vi "MICSD Config.vi"(8 "error in (no error)":errorcluster, 9 "Function":enum16{"Write Config", "Read Config"}(ring), 10 "MICS_Config_In":T1={"ConfigFlags"=0, "ImplantID"=1193046, "CompanyID"=1, "Normal_Comm"={"RF_Channel"=4, "UserData"=0, "TX_Mod"=0, "RX_Mod"=0, "RX_BlockSize"=15, "BlockPerPack"=31, "TX_BlockSize"=15}, "Emerg_Comm"={"RF_Channel"=4, "UserData"=0, "TX_Mod"=0, "RX_Mod"=0, "TX_BlockSize"=15, "BlockPerPack"=31, "RX_BlockSize"=15}, "ImplantRev"=5, "245TX_PowerCal"=0, "245TX_Power"=10, "CCA_RSSI_Thresholds"={"ch0"=2650, "ch1"=2650, "ch2"=2650, "ch3"=2650, "ch4"=2650, "ch5"=2650, "ch6"=2650, "ch7"=2650, "ch8"=2650, "ch9"=2650}} {"ConfigFlags" format="%02x"; "ImplantID" format="%06x"; "CompanyID" format="%02x"; "Normal_Comm"."TX_BlockSize" items=["2"=2, "3"=3, "4"=4, "5"=5, "6"=6, "7"=7, "8"=8, "9"=9, "10"=10, "11"=11, "12"=12, "13"=13, "14"=14, "15"=15, "16"=16, "17"=17, "18"=18, "19"=19, "20"=20, "21"=21, "22"=22, "23"=23, "24"=24, "25"=25, "26"=26, "27"=27, "28"=28, "29"=29, "30"=30, "31"=31]; "Normal_Comm"."RF_Channel" items=["0", "1", "2", "3", "4", "5", "6", "7", "8", "9", "10", "11"]; "Normal_Comm"."UserData" items=["0 - 000"=0, "1 - 001"=16, "2 - 010"=32, "3 - 011"=48, "4 - 100"=64, "5 - 101"=80, "6 - 110"=96, "7 - 111"=112]; "Normal_Comm"."TX_Mod" items=["2FSK-FB"=0, "2FSK"=2, "4FSK"=3]; "Normal_Comm"."RX_Mod" items=["2FSK-FB"=0, "2FSK"=8, "4FSK"=12]; "Normal_Comm"."RX_BlockSize" items=["2"=2, "3"=3, "4"=4, "5"=5, "6"=6, "7"=7, "8"=8, "9"=9, "10"=10, "11"=11, "12"=12, "13"=13, "14"=14, "15"=15, "16"=16, "17"=17, "18"=18, "19"=19, "20"=20, "21"=21, "22"=22, "23"=23, "24"=24, "25"=25, "26"=26, "27"=27, "28"=28, "29"=29, "30"=30, "31"=31]; "Normal_Comm"."BlockPerPack" items=["1"=1, "2"=2, "3"=3, "4"=4, "5"=5, "6"=6, "7"=7, "8"=8, "9"=9, "10"=10, "11"=11, "12"=12, "13"=13, "14"=14, "15"=15, "16"=16, "17"=17, "18"=18, "19"=19, "20"=20, "21"=21, "22"=22, "23"=23, "24"=24, "25"=25, "26"=26, "27"=27, "28"=28, "29"=29, "30"=30, "31"=31]; "Emerg_Comm"."RX_BlockSize" items=["2"=2, "3"=3, "4"=4, "5"=5, "6"=6, "7"=7, "8"=8, "9"=9, "10"=10, "11"=11, "12"=12, "13"=13, "14"=14, "15"=15, "16"=16, "17"=17, "18"=18, "19"=19, "20"=20, "21"=21, "22"=22, "23"=23, "24"=24, "25"=25, "26"=26, "27"=27, "28"=28, "29"=29, "30"=30, "31"=31]; "Emerg_Comm"."RF_Channel" items=["0", "1", "2", "3", "4", "5", "6", "7", "8", "9"]; "Emerg_Comm"."UserData" items=["0 - 000"=0, "1 - 001"=16, "2 - 010"=32, "3 - 011"=48, "4 - 100"=64, "5 - 101"=80, "6 - 110"=96, "7 - 111"=112]; "Emerg_Comm"."TX_Mod" items=["2FSK-FB"=0, "2FSK"=2, "4FSK"=3]; "Emerg_Comm"."RX_Mod" items=["2FSK-FB"=0, "2FSK"=8, "4FSK"=12]; "Emerg_Comm"."TX_BlockSize" items=["2"=2, "3"=3, "4"=4, "5"=5, "6"=6, "7"=7, "8"=8, "9"=9, "10"=10, "11"=11, "12"=12, "13"=13, "14"=14, "15"=15, "16"=16, "17"=17, "18"=18, "19"=19, "20"=20, "21"=21, "22"=22, "23"=23, "24"=24, "25"=25, "26"=26, "27"=27, "28"=28, "29"=29, "30"=30, "31"=31]; "Emerg_Comm"."BlockPerPack" items=["1"=1, "2"=2, "3"=3, "4"=4, "5"=5, "6"=6, "7"=7, "8"=8, "9"=9, "10"=10, "11"=11, "12"=12, "13"=13, "14"=14, "15"=15, "16"=16, "17"=17, "18"=18, "19"=19, "20"=20, "21"=21, "22"=22, "23"=23, "24"=24, "25"=25, "26"=26, "27"=27, "28"=28, "29"=29, "30"=30, "31"=31]; "ImplantRev" items=["ZL70100"=0, "ZL70101"=1, "ZL70102"=4, "ZL70103"=5]; "245TX_PowerCal" items=["-29"=-29, "-4"=-4, "-2"=-2, "0"=0, "2"=2, "4"=4, "6"=6, "8"=8, "10"=10, "12"=12, "14"=14, "16"=16, "18"=18, "20"=20, "22"=22, "24"=24, "26"=26, "27"=27]; "245TX_Power" items=["-29"=-29, "-4"=-4, "-2"=-2, "0"=0, "2"=2, "4"=4, "6"=6, "8"=8, "10"=10, "12"=12, "14"=14, "16"=16, "18"=18, "20"=20, "22"=22, "24"=24, "26"=26, "27"=27]}, 11 "VISA Resource Name":refnum<visa-resource-name>) -> (0 "error out":errorcluster, 1 "Reply Header":u8[](array[numeric]), 3 "dup VISA Resource Name":refnum<visa-resource-name>)   [LabVIEW 2020]
uses:
  <vilib>/Instr/_visa.llb/VISA Configure Serial Port (Instr).vi
panel:
  out "Written Config":u8[](array[numeric]) format="%02x"
  out "MICS_Config_OUT":T1={"ConfigFlags"=0, "ImplantID"=1048576, "CompanyID"=187, "Normal_Comm"={"RF_Channel"=4, "UserData"=0, "TX_Mod"=2, "RX_Mod"=8, "RX_BlockSize"=15, "BlockPerPack"=31, "TX_BlockSize"=15}, "Emerg_Comm"={"RF_Channel"=4, "UserData"=0, "TX_Mod"=2, "RX_Mod"=8, "TX_BlockSize"=15, "BlockPerPack"=31, "RX_BlockSize"=15}, "ImplantRev"=4, "245TX_PowerCal"=0, "245TX_Power"=10, "CCA_RSSI_Thresholds"={"ch0"=2650, "ch1"=2650, "ch2"=2650, "ch3"=2650, "ch4"=2650, "ch5"=2650, "ch6"=2650, "ch7"=2650, "ch8"=2650, "ch9"=2650}} {"ConfigFlags" format="%02x"; "ImplantID" format="%06x"; "CompanyID" format="%02x"; "Normal_Comm"."TX_BlockSize" items=["2"=2, "3"=3, "4"=4, "5"=5, "6"=6, "7"=7, "8"=8, "9"=9, "10"=10, "11"=11, "12"=12, "13"=13, "14"=14, "15"=15, "16"=16, "17"=17, "18"=18, "19"=19, "20"=20, "21"=21, "22"=22, "23"=23, "24"=24, "25"=25, "26"=26, "27"=27, "28"=28, "29"=29, "30"=30, "31"=31]; "Normal_Comm"."RF_Channel" items=["0", "1", "2", "3", "4", "5", "6", "7", "8", "9"]; "Normal_Comm"."UserData" items=["0 - 000"=0, "1 - 001"=16, "2 - 010"=32, "3 - 011"=48, "4 - 100"=64, "5 - 101"=80, "6 - 110"=96, "7 - 111"=112]; "Normal_Comm"."TX_Mod" items=["2FSK-FB"=0, "2FSK"=2, "4FSK"=3]; "Normal_Comm"."RX_Mod" items=["2FSK-FB"=0, "2FSK"=8, "4FSK"=12]; "Normal_Comm"."RX_BlockSize" items=["2"=2, "3"=3, "4"=4, "5"=5, "6"=6, "7"=7, "8"=8, "9"=9, "10"=10, "11"=11, "12"=12, "13"=13, "14"=14, "15"=15, "16"=16, "17"=17, "18"=18, "19"=19, "20"=20, "21"=21, "22"=22, "23"=23, "24"=24, "25"=25, "26"=26, "27"=27, "28"=28, "29"=29, "30"=30, "31"=31]; "Normal_Comm"."BlockPerPack" items=["1"=1, "2"=2, "3"=3, "4"=4, "5"=5, "6"=6, "7"=7, "8"=8, "9"=9, "10"=10, "11"=11, "12"=12, "13"=13, "14"=14, "15"=15, "16"=16, "17"=17, "18"=18, "19"=19, "20"=20, "21"=21, "22"=22, "23"=23, "24"=24, "25"=25, "26"=26, "27"=27, "28"=28, "29"=29, "30"=30, "31"=31]; "Emerg_Comm"."RX_BlockSize" items=["2"=2, "3"=3, "4"=4, "5"=5, "6"=6, "7"=7, "8"=8, "9"=9, "10"=10, "11"=11, "12"=12, "13"=13, "14"=14, "15"=15, "16"=16, "17"=17, "18"=18, "19"=19, "20"=20, "21"=21, "22"=22, "23"=23, "24"=24, "25"=25, "26"=26, "27"=27, "28"=28, "29"=29, "30"=30, "31"=31]; "Emerg_Comm"."RF_Channel" items=["0", "1", "2", "3", "4", "5", "6", "7", "8", "9"]; "Emerg_Comm"."UserData" items=["0 - 000"=0, "1 - 001"=16, "2 - 010"=32, "3 - 011"=48, "4 - 100"=64, "5 - 101"=80, "6 - 110"=96, "7 - 111"=112]; "Emerg_Comm"."TX_Mod" items=["2FSK-FB"=0, "2FSK"=2, "4FSK"=3]; "Emerg_Comm"."RX_Mod" items=["2FSK-FB"=0, "2FSK"=8, "4FSK"=12]; "Emerg_Comm"."TX_BlockSize" items=["2"=2, "3"=3, "4"=4, "5"=5, "6"=6, "7"=7, "8"=8, "9"=9, "10"=10, "11"=11, "12"=12, "13"=13, "14"=14, "15"=15, "16"=16, "17"=17, "18"=18, "19"=19, "20"=20, "21"=21, "22"=22, "23"=23, "24"=24, "25"=25, "26"=26, "27"=27, "28"=28, "29"=29, "30"=30, "31"=31]; "Emerg_Comm"."BlockPerPack" items=["1"=1, "2"=2, "3"=3, "4"=4, "5"=5, "6"=6, "7"=7, "8"=8, "9"=9, "10"=10, "11"=11, "12"=12, "13"=13, "14"=14, "15"=15, "16"=16, "17"=17, "18"=18, "19"=19, "20"=20, "21"=21, "22"=22, "23"=23, "24"=24, "25"=25, "26"=26, "27"=27, "28"=28, "29"=29, "30"=30, "31"=31]; "ImplantRev" items=["ZL70100"=0, "ZL70101"=1, "ZL70102"=4, "ZL70103"=5]; "245TX_PowerCal" items=["-29"=-29, "-4"=-4, "-2"=-2, "0"=0, "2"=2, "4"=4, "6"=6, "8"=8, "10"=10, "12"=12, "14"=14, "16"=16, "18"=18, "20"=20, "22"=22, "24"=24, "26"=26, "27"=27]; "245TX_Power" items=["-29"=-29, "-4"=-4, "-2"=-2, "0"=0, "2"=2, "4"=4, "6"=6, "8"=8, "10"=10, "12"=12, "14"=14, "16"=16, "18"=18, "20"=20, "22"=22, "24"=24, "26"=26, "27"=27]}
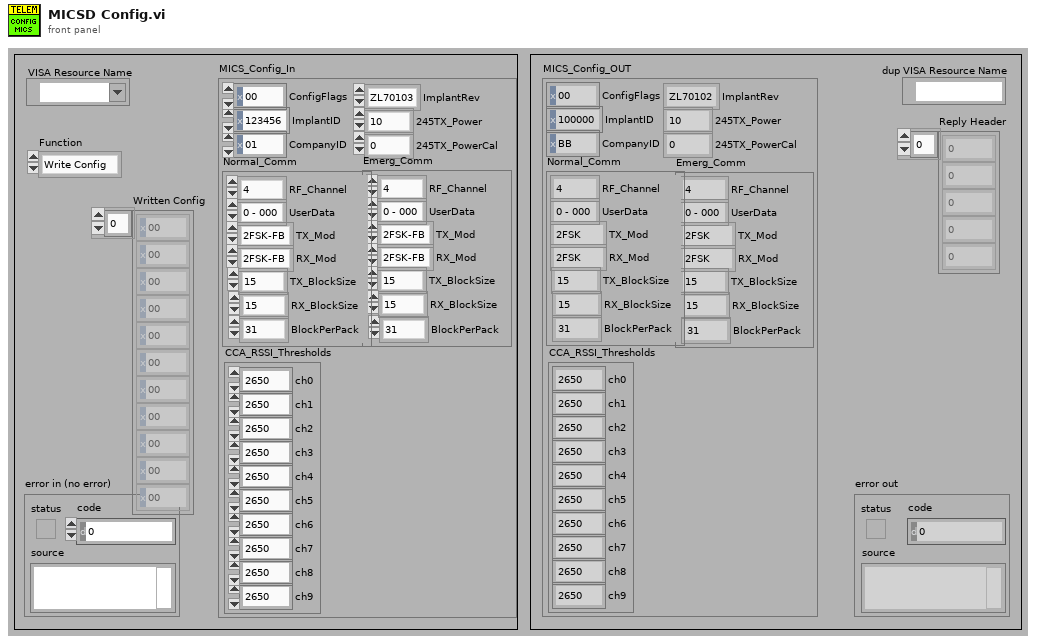
[diagram p1: front panel]
types:
  T1 = cluster{"ConfigFlags":u8, "ImplantID":u32, "CompanyID":u8, "Normal_Comm":cluster{"RF_Channel":u8, "UserData":u8, "TX_Mod":u8, "RX_Mod":u8, "RX_BlockSize":u8, "BlockPerPack":u8, "TX_BlockSize":u8}, "Emerg_Comm":cluster{"RF_Channel":u8, "UserData":u8, "TX_Mod":u8, "RX_Mod":u8, "TX_BlockSize":u8, "BlockPerPack":u8, "RX_BlockSize":u8}, "ImplantRev":u8, "245TX_PowerCal":i8, "245TX_Power":i8, "CCA_RSSI_Thresholds":cluster{"ch0":u16, "ch1":u16, "ch2":u16, "ch3":u16, "ch4":u16, "ch5":u16, "ch6":u16, "ch7":u16, "ch8":u16, "ch9":u16}}
  T2 = cluster{"Command Token":u8, "Length":u16, "Pack Data":u8[]}
  T3 = cluster{"RF_Channel":u8, "UserData":u8, "TX_Mod":u8, "RX_Mod":u8, "RX_BlockSize":u8, "BlockPerPack":u8, "TX_BlockSize":u8}
  T4 = cluster{"RF_Channel":u8, "UserData":u8, "TX_Mod":u8, "RX_Mod":u8, "TX_BlockSize":u8, "BlockPerPack":u8, "RX_BlockSize":u8}
  T5 = cluster{"ch0":u16, "ch1":u16, "ch2":u16, "ch3":u16, "ch4":u16, "ch5":u16, "ch6":u16, "ch7":u16, "ch8":u16, "ch9":u16}
  T6 = cluster{"Read Data[0]":u8, "Read Data[1]":u8, "Read Data[2]":u8, "Read Data[3]":u8, "Read Data[4]":u8, "Read Data[5]":u8, "Read Data[6]":u8, "Read Data[7]":u8, "Read Data[8]":u8, "Read Data[9]":u8, "Read Data[10]":u8, "Read Data[11]":u8, "Read Data[12]":u8, "Read Data[13]":u8, "Read Data[14]":u8, "Read Data[15]":u8, "Read Data[16]":u8, "Read Data[17]":u8, "Read Data[18]":u8, "Read Data[19]":u8, "Read Data[20]":u8, "Read Data[21]":u8, "Read Data[22]":u8, "Read Data[23]":u8, "Read Data[24]":u8, "Read Data[25]":u8, "Read Data[26]":u8, "Read Data[27]":u8, "Read Data[28]":u8, "Read Data[29]":u8, "Read Data[30]":u8, "Read Data[31]":u8, "Read Data[32]":u8, "Read Data[33]":u8, "Read Data[34]":u8, "Read Data[35]":u8, "Read Data[36]":u8, "Read Data[37]":u8, "Read Data[38]":u8, "Read Data[39]":u8, "Read Data[40]":u8, "Read Data[41]":u8}
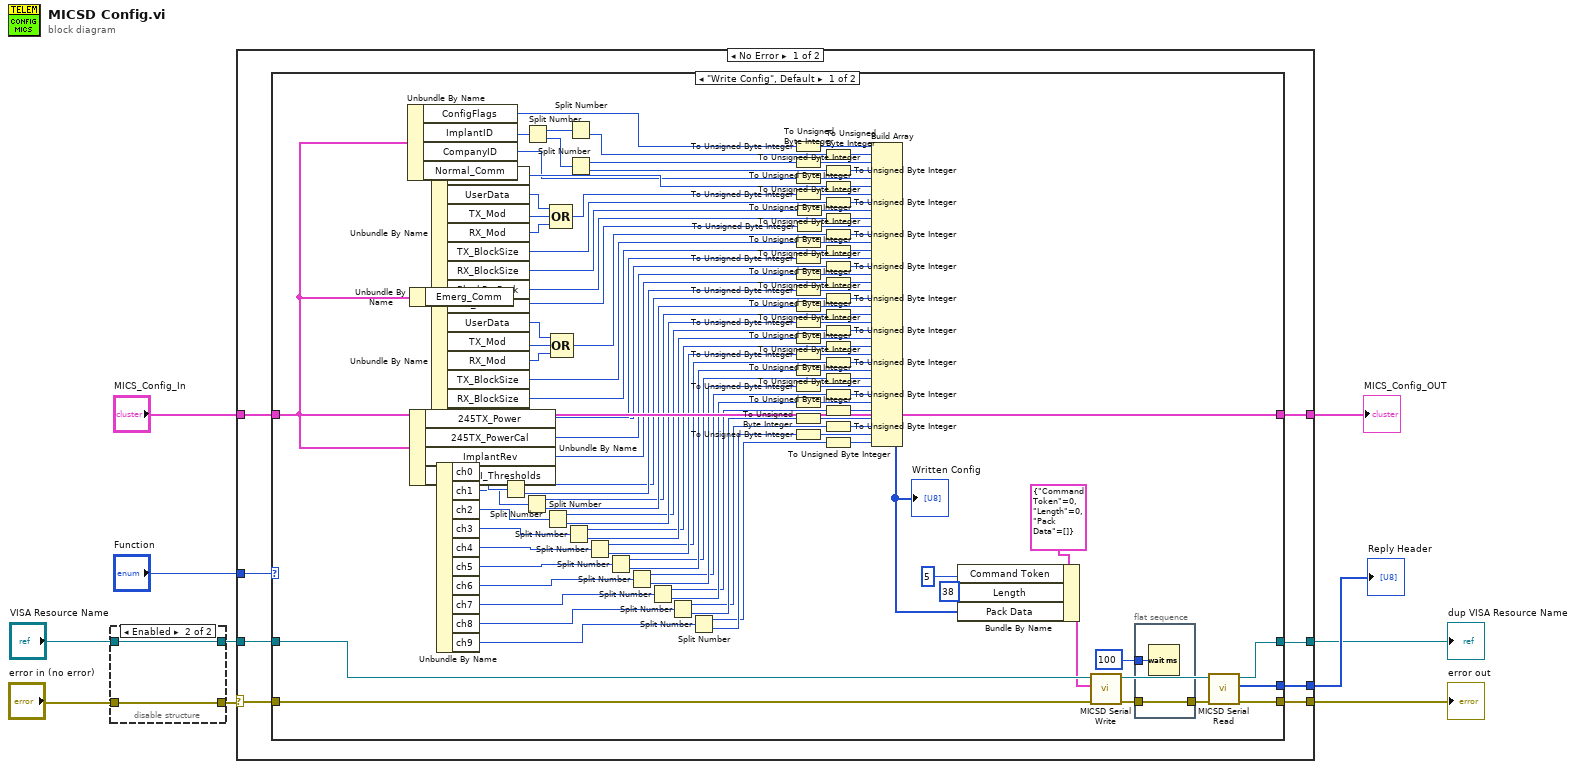
[diagram p0: block diagram]
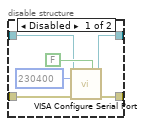
[diagram p2: hidden frame]
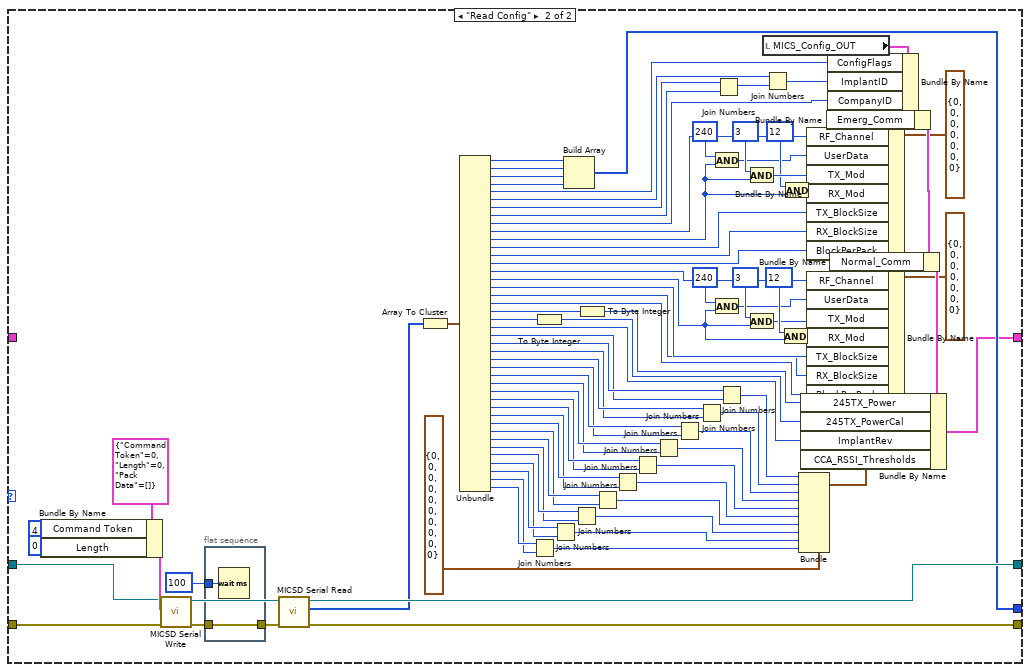
[diagram p3: hidden frame]
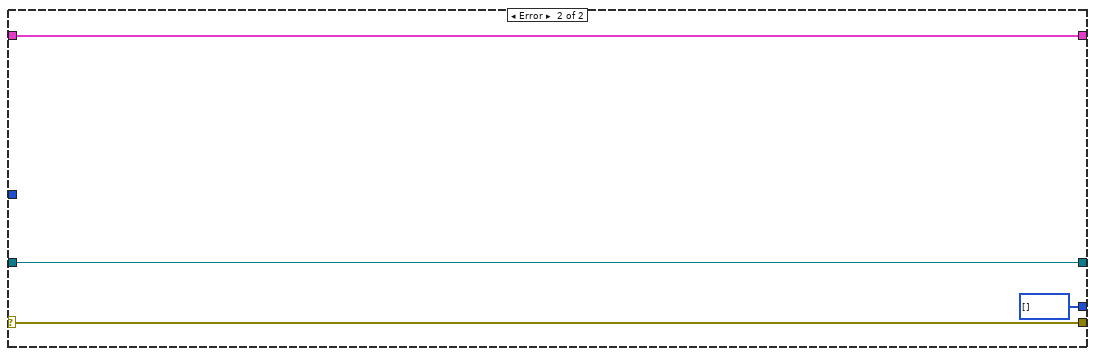
[diagram p4: hidden frame]
diagram:
  n1 = disable-structure shown="Enabled" {
    disable-tunnel: [w14 w17] -> w7
    disable-tunnel: "error in (no error)" -> [w13 w17]
    disable-tunnel: "VISA Resource Name" -> [w12 w18]
    disable-tunnel: [w11 w18] -> w4
    frame Disabled {
      n2 = call-poly "VISA Configure Serial Port"("VISA resource name"=w12, "Enable Termination\nChar (T)"=FALSE ("Enable Termination\nChar (T)"), "baud rate (9600)"=u32 230400, "error in (no error)"=w13) -> ("VISA resource name out"=w11:refnum<visa-resource-name>, "error out"=w14:errorcluster)  [unwired: 10 in]
    }
    frame Enabled {
    }
  }
  n3 = case shown="No Error" w7 {
    selector: w7 -> [w26 w241]
    tunnel: w4 -> [w25 w240]
    tunnel: [w22 w241] -> w2
    tunnel: [w23 w240] -> w3
    tunnel: "MICS_Config_In" -> [w24 w239]
    tunnel: "Function" -> [w21 _]
    tunnel: [w20 u8[] [] ("Read Data")] -> w8
    tunnel: [w19 w239] -> w1
    frame No Error {
      n4 = case shown="\"Write Config\", Default" w21 {
        tunnel: w26 -> [w139 w227]
        tunnel: w25 -> [w136 w224]
        tunnel: w24 -> [w70 _]
        tunnel: [w75 w225] -> w23
        tunnel: [w76 w226] -> w22
        tunnel: [w73 w204] -> w20
        tunnel: [w70 w144] -> w19
        frame "Write Config", Default {
          n5 = Unbundle By Name(w70) -> ("ConfigFlags"=w132:u8, "ImplantID"=w131:u32, "CompanyID"=w123:u8, "Normal_Comm"=w135:T3)
          n6 = Unbundle By Name(w70) -> ("Emerg_Comm"=w134:T4)
          n7 = Unbundle By Name(w70) -> ("245TX_Power"=w53:i8, "245TX_PowerCal"=w52:i8, "ImplantRev"=w51:u8, "CCA_RSSI_Thresholds"=w133:T5)
          n8 = Unbundle By Name(w135) -> ("RF_Channel"=w124:u8, "UserData"=w27:u8, "TX_Mod"=w68:u8, "RX_Mod"=w67:u8, "TX_BlockSize"=w122:u8, "RX_BlockSize"=w60:u8, "BlockPerPack"=w59:u8)
          n9 = Unbundle By Name(w134) -> ("RF_Channel"=w58:u8, "UserData"=w28:u8, "TX_Mod"=w65:u8, "RX_Mod"=w64:u8, "TX_BlockSize"=w56:u8, "RX_BlockSize"=w55:u8, "BlockPerPack"=w54:u8)
          n10 = Unbundle By Name(w133) -> ("ch0"=w87:u16, "ch1"=w86:u16, "ch2"=w85:u16, "ch3"=w84:u16, "ch4"=w83:u16, "ch5"=w82:u16, "ch6"=w81:u16, "ch7"=w80:u16, "ch8"=w79:u16, "ch9"=w78:u16)
          n11 = Split Number(x=w87) -> (hi(x)=w49:u8, lo(x)=w50:u8)
          n12 = Split Number(x=w86) -> (hi(x)=w47:u8, lo(x)=w48:u8)
          n13 = Split Number(x=w131) -> (hi(x)=w69:u16, lo(x)=w130:u16)
          n14 = Split Number(x=w85) -> (hi(x)=w45:u8, lo(x)=w46:u8)
          n15 = Compound Arithmetic op=OR(w27, w68, w67) -> (w66:u8)
          n16 = Compound Arithmetic op=OR(w28, w65, w64) -> (w57:u8)
          n17 = Split Number(x=w84) -> (hi(x)=w43:u8, lo(x)=w44:u8)
          n18 = Split Number(x=w69) -> (lo(x)=w61:u8)  [unwired: 1 out]
          n19 = Split Number(x=w130) -> (hi(x)=w62:u8, lo(x)=w63:u8)
          n20 = Split Number(x=w83) -> (hi(x)=w41:u8, lo(x)=w42:u8)
          n21 = Split Number(x=w82) -> (hi(x)=w39:u8, lo(x)=w40:u8)
          n22 = Split Number(x=w81) -> (hi(x)=w37:u8, lo(x)=w38:u8)
          n23 = Split Number(x=w80) -> (hi(x)=w35:u8, lo(x)=w36:u8)
          n24 = Split Number(x=w79) -> (hi(x)=w33:u8, lo(x)=w34:u8)
          n25 = Split Number(x=w78) -> (hi(x)=w31:u8, lo(x)=w32:u8)
          n26 = To Unsigned Byte Integer(number=w132) -> (unsigned 8bit integer=w129:u8)
          n27 = To Unsigned Byte Integer(number=w62) -> (unsigned 8bit integer=w127:u8)
          n28 = To Unsigned Byte Integer(number=w123) -> (unsigned 8bit integer=w125:u8)
          n29 = To Unsigned Byte Integer(number=w66) -> (unsigned 8bit integer=w120:u8)
          n30 = To Unsigned Byte Integer(number=w56) -> (unsigned 8bit integer=w114:u8)
          n31 = To Unsigned Byte Integer(number=w54) -> (unsigned 8bit integer=w112:u8)
          n32 = To Unsigned Byte Integer(number=w52) -> (unsigned 8bit integer=w110:u8)
          n33 = To Unsigned Byte Integer(number=w50) -> (unsigned 8bit integer=w108:u8)
          n34 = To Unsigned Byte Integer(number=w48) -> (unsigned 8bit integer=w106:u8)
          n35 = To Unsigned Byte Integer(number=w46) -> (unsigned 8bit integer=w104:u8)
          n36 = To Unsigned Byte Integer(number=w44) -> (unsigned 8bit integer=w102:u8)
          n37 = To Unsigned Byte Integer(number=w42) -> (unsigned 8bit integer=w97:u8)
          n38 = To Unsigned Byte Integer(number=w40) -> (unsigned 8bit integer=w95:u8)
          n39 = To Unsigned Byte Integer(number=w38) -> (unsigned 8bit integer=w93:u8)
          n40 = To Unsigned Byte Integer(number=w36) -> (unsigned 8bit integer=w91:u8)
          n41 = To Unsigned Byte Integer(number=w34) -> (unsigned 8bit integer=w89:u8)
          n42 = To Unsigned Byte Integer(number=w32) -> (unsigned 8bit integer=w30:u8)
          n43 = To Unsigned Byte Integer(number=w60) -> (unsigned 8bit integer=w118:u8)
          n44 = To Unsigned Byte Integer(number=w58) -> (unsigned 8bit integer=w116:u8)
          n45 = To Unsigned Byte Integer(number=w61) -> (unsigned 8bit integer=w128:u8)
          n46 = To Unsigned Byte Integer(number=w63) -> (unsigned 8bit integer=w126:u8)
          n47 = To Unsigned Byte Integer(number=w124) -> (unsigned 8bit integer=w121:u8)
          n48 = To Unsigned Byte Integer(number=w122) -> (unsigned 8bit integer=w119:u8)
          n49 = To Unsigned Byte Integer(number=w59) -> (unsigned 8bit integer=w117:u8)
          n50 = To Unsigned Byte Integer(number=w57) -> (unsigned 8bit integer=w115:u8)
          n51 = To Unsigned Byte Integer(number=w55) -> (unsigned 8bit integer=w113:u8)
          n52 = To Unsigned Byte Integer(number=w53) -> (unsigned 8bit integer=w111:u8)
          n53 = To Unsigned Byte Integer(number=w51) -> (unsigned 8bit integer=w109:u8)
          n54 = To Unsigned Byte Integer(number=w49) -> (unsigned 8bit integer=w107:u8)
          n55 = To Unsigned Byte Integer(number=w47) -> (unsigned 8bit integer=w105:u8)
          n56 = To Unsigned Byte Integer(number=w45) -> (unsigned 8bit integer=w103:u8)
          n57 = To Unsigned Byte Integer(number=w43) -> (unsigned 8bit integer=w101:u8)
          n58 = To Unsigned Byte Integer(number=w41) -> (unsigned 8bit integer=w96:u8)
          n59 = To Unsigned Byte Integer(number=w39) -> (unsigned 8bit integer=w94:u8)
          n60 = To Unsigned Byte Integer(number=w37) -> (unsigned 8bit integer=w92:u8)
          n61 = To Unsigned Byte Integer(number=w35) -> (unsigned 8bit integer=w90:u8)
          n62 = To Unsigned Byte Integer(number=w33) -> (unsigned 8bit integer=w88:u8)
          n63 = To Unsigned Byte Integer(number=w31) -> (unsigned 8bit integer=w29:u8)
          n64 = Build Array(w129, w128, w127, w126, w125, w121, w120, w119, w118, w117, w116, w115, w114, w113, w112, w111, w110, w109, w108, w107, w106, w105, w104, w103, w102, w101, w97, w96, w95, w94, w93, w92, w91, w90, w89, w88, w30, w29) -> (w98:u8[])
          "Written Config" <- w98
          n65 = Bundle By Name(cluster=T2 {"Command Token"=0, "Length"=0, "Pack Data"=[]} ("Write Data"), "Command Token"=u8 5, "Length"=u16 38, "Pack Data"=w98) -> (w100:T2)
          n66 = call "MICSD Serial Write.vi"("error in (no error)"=w139, "Write Data"=w100, "VISA Resource Name"=w136) -> ("error out"=w138:errorcluster, "DUP Visa Resource Name"=w74:refnum<visa-resource-name>)  [unwired: 7 in]
          n67 = flat-sequence {
            tunnel: w138 -> [w141]
            tunnel: [w141] -> w77
            tunnel: 100 -> [w140]
            frame #0 {
              n68 = Wait (ms)(milliseconds to wait=w140) -> ()  [unwired: 1 out]
            }
          }
          n69 = call "MICSD Serial Read.vi"("error in (no error)"=w77, "VISA Resource Name"=w74) -> ("error out"=w76:errorcluster, "Read Data"=w73:u8[], "DUP Visa Resource Name"=w75:refnum<visa-resource-name>)  [unwired: 7 in]
        }
        frame "Read Config" {
          n70 = Bundle By Name(cluster=T2 {"Command Token"=0, "Length"=0, "Pack Data"=[]} ("Write Data"), "Command Token"=u8 4, "Length"=u16 0) -> (w233:T2)
          n71 = call "MICSD Serial Write.vi"("error in (no error)"=w227, "Write Data"=w233, "VISA Resource Name"=w224) -> ("error out"=w235:errorcluster, "DUP Visa Resource Name"=w230:refnum<visa-resource-name>)  [unwired: 7 in]
          n72 = flat-sequence {
            tunnel: w235 -> [w237]
            tunnel: [w237] -> w231
            tunnel: 100 -> [w236]
            frame #0 {
              n73 = Wait (ms)(milliseconds to wait=w236) -> ()  [unwired: 1 out]
            }
          }
          n74 = call "MICSD Serial Read.vi"("error in (no error)"=w231, "VISA Resource Name"=w230) -> ("error out"=w226:errorcluster, "Read Data"=w223:u8[], "DUP Visa Resource Name"=w225:refnum<visa-resource-name>)  [unwired: 7 in]
          n75 = Array To Cluster(array=w223) -> (cluster=w197:T6)
          n76 = Unbundle(w197) -> ("Read Data[0]"=w164:u8, "Read Data[1]"=w165:u8, "Read Data[2]"=w166:u8, "Read Data[3]"=w167:u8, "Read Data[4]"=w168:u8, "Read Data[5]"=w169:u8, "Read Data[6]"=w170:u8, "Read Data[7]"=w171:u8, "Read Data[8]"=w172:u8, "Read Data[9]"=w173:u8, "Read Data[10]"=w158:u8, "Read Data[11]"=w154:u8, "Read Data[12]"=w153:u8, "Read Data[13]"=w152:u8, "Read Data[14]"=w149:u8, "Read Data[15]"=w148:u8, "Read Data[16]"=w147:u8, "Read Data[17]"=w146:u8, "Read Data[18]"=w145:u8, "Read Data[19]"=w174:u8, "Read Data[20]"=w175:u8, "Read Data[21]"=w176:u8, "Read Data[22]"=w177:u8, "Read Data[23]"=w178:u8, "Read Data[24]"=w179:u8, "Read Data[25]"=w180:u8, "Read Data[26]"=w181:u8, "Read Data[27]"=w182:u8, "Read Data[28]"=w183:u8, "Read Data[29]"=w184:u8, "Read Data[30]"=w185:u8, "Read Data[31]"=w186:u8, "Read Data[32]"=w187:u8, "Read Data[33]"=w188:u8, "Read Data[34]"=w189:u8, "Read Data[35]"=w190:u8, "Read Data[36]"=w191:u8, "Read Data[37]"=w192:u8, "Read Data[38]"=w193:u8, "Read Data[39]"=w194:u8, "Read Data[40]"=w195:u8, "Read Data[41]"=w196:u8)
          n77 = Join Numbers(hi=w196, lo=w195) -> ((hi.lo)=w205:u16)
          n78 = To Byte Integer(number=w175) -> (8bit integer=w142:i8)
          n79 = Join Numbers(hi=w194, lo=w193) -> ((hi.lo)=w206:u16)
          n80 = Build Array(w164, w165, w166, w167) -> (w204:u8[])
          n81 = Join Numbers(hi=w192, lo=w191) -> ((hi.lo)=w207:u16)
          n82 = To Byte Integer(number=w174) -> (8bit integer=w143:i8)
          n83 = Join Numbers(hi=w190, lo=w189) -> ((hi.lo)=w208:u16)
          n84 = Join Numbers(hi=w188, lo=w187) -> ((hi.lo)=w209:u16)
          n85 = Join Numbers(hi=w186, lo=w185) -> ((hi.lo)=w210:u16)
          n86 = Join Numbers(hi=w184, lo=w183) -> ((hi.lo)=w211:u16)
          n87 = Join Numbers(hi=w182, lo=w181) -> ((hi.lo)=w212:u16)
          n88 = Join Numbers(hi=w180, lo=w179) -> ((hi.lo)=w213:u16)
          n89 = And(x=u8 240 ("Command Token"), y=w158) -> (x .and. y?=w162:u8)
          n90 = And(x=u8 240 ("Command Token"), y=w148) -> (x .and. y?=w159:u8)
          n91 = Join Numbers(hi=w170, lo=w171) -> ((hi.lo)=w222:u16)
          n92 = Join Numbers(hi=w178, lo=w177) -> ((hi.lo)=w214:u16)
          n93 = And(x=u8 3 ("Command Token"), y=w158) -> (x .and. y?=w220:u8)
          n94 = And(x=u8 3 ("Command Token"), y=w148) -> (x .and. y?=w199:u8)
          n95 = local read "MICS_Config_OUT"() -> (w163:T1)
          n96 = Join Numbers(hi=w169, lo=w222) -> ((hi.lo)=w221:u32)
          n97 = And(x=u8 12 ("Command Token"), y=w148) -> (x .and. y?=w198:u8)
          n98 = And(x=u8 12 ("Command Token"), y=w158) -> (x .and. y?=w219:u8)
          n99 = Bundle(cluster=T5 {"ch0"=0, "ch1"=0, "ch2"=0, "ch3"=0, "ch4"=0, "ch5"=0, "ch6"=0, "ch7"=0, "ch8"=0, "ch9"=0} ("CCA_RSSI_Thresholds"), "ch0"=w214, "ch1"=w213, "ch2"=w212, "ch3"=w211, "ch4"=w210, "ch5"=w209, "ch6"=w208, "ch7"=w207, "ch8"=w206, "ch9"=w205) -> (w216:T5)
          n100 = Bundle By Name(cluster=T4 {"RF_Channel"=0, "UserData"=0, "TX_Mod"=0, "RX_Mod"=0, "TX_BlockSize"=0, "BlockPerPack"=0, "RX_BlockSize"=0} ("Emerg_Comm"), "RF_Channel"=w173, "UserData"=w162, "TX_Mod"=w220, "RX_Mod"=w219, "TX_BlockSize"=w154, "RX_BlockSize"=w153, "BlockPerPack"=w152) -> (w155:T4)
          n101 = Bundle By Name(cluster=T3 {"RF_Channel"=0, "UserData"=0, "TX_Mod"=0, "RX_Mod"=0, "RX_BlockSize"=0, "BlockPerPack"=0, "TX_BlockSize"=0} ("Normal_Comm"), "RF_Channel"=w149, "UserData"=w159, "TX_Mod"=w199, "RX_Mod"=w198, "TX_BlockSize"=w147, "RX_BlockSize"=w146, "BlockPerPack"=w145) -> (w150:T3)
          n102 = Bundle By Name(cluster=w163, "ConfigFlags"=w168, "ImplantID"=w221, "CompanyID"=w172) -> (w157:T1)
          n103 = Bundle By Name(cluster=w157, "Emerg_Comm"=w155) -> (w203:T1)
          n104 = Bundle By Name(cluster=w203, "Normal_Comm"=w150) -> (w202:T1)
          n105 = Bundle By Name(cluster=w202, "245TX_Power"=w143, "245TX_PowerCal"=w142, "ImplantRev"=w176, "CCA_RSSI_Thresholds"=w216) -> (w144:T1)
        }
      }
    }
    frame Error {
    }
  }
  "error out" <- w2
  "dup VISA Resource Name" <- w3
  "Reply Header" <- w8
  "MICS_Config_OUT" <- w1
